vi "string_conversion.vi"(11 "FName":u64[](array[numeric])) -> (3 "string":string)   [LabVIEW 2014]
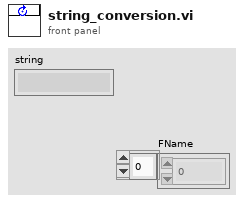
[diagram p1: front panel]
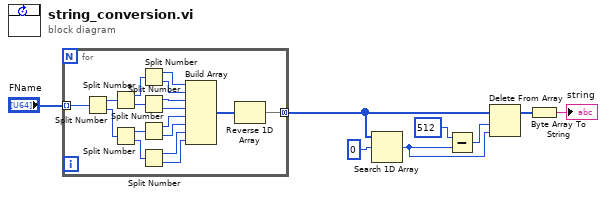
[diagram p0: block diagram]
diagram:
  n1 = for {
    tunnel: "FName" -> [w25] mode=indexing
    tunnel: [w9] -> w1 mode=concatenating
    n2 = Split Number(x=w25) -> (hi(x)=w24:u32, lo(x)=w23:u32)
    n3 = Split Number(x=w24) -> (hi(x)=w22:u16, lo(x)=w21:u16)
    n4 = Split Number(x=w23) -> (hi(x)=w20:u16, lo(x)=w19:u16)
    n5 = Split Number(x=w22) -> (hi(x)=w18:u8, lo(x)=w17:u8)
    n6 = Split Number(x=w21) -> (hi(x)=w16:u8, lo(x)=w15:u8)
    n7 = Split Number(x=w20) -> (hi(x)=w14:u8, lo(x)=w13:u8)
    n8 = Split Number(x=w19) -> (hi(x)=w12:u8, lo(x)=w11:u8)
    n9 = Build Array(w18, w17, w16, w15, w14, w13, w12, w11) -> (w10:u8[])
    n10 = Reverse 1D Array(array=w10) -> (reversed array=w9:u8[])
  }
  n11 = Search 1D Array(1D array=w1, element=u8 0 ("元素")) -> (index of element=w7:i32)  [unwired: 1 in]
  n12 = Subtract(x=512, y=w7) -> (x-y=w6:i32)
  n13 = Delete From Array(array=w1, length=w6, index=w7) -> (array with subset deleted=w4:u8[])  [unwired: 1 out]
  n14 = Byte Array To String(unsigned byte array=w4) -> (string=→"string":string)
